vi "Compare Two Paths - Path2 Array.vi"(4 "path2":path[](array[path]), 5 "path1":path) -> (0 "any different types?":bool, 1 "relative path from 1 to 2":path[](array[path]), 2 "common path":path[](array[path]))   [LabVIEW 2020, in "openg_file.lvlib"]
doc: "Compare Two Paths.vi - Compares two paths and if the paths are the same type (both absolute or both relative), the relative path between them is returned."
uses:
  openg_file.lvlib
panel:
  # "Compare Two Paths - Path2 Array.vi\n\nCompares two paths and if the paths are the same type (both absolute or both relative), the relative path between them is returned.\n\nPlease visit http://www.OpenG.org to learn about the\nOpen Source LabVIEW software movement.\n\nNOTICE -- YOU MUST LEAVE THIS NOTICE IN PLACE.  PER THE TERMS OF THE LICENSE BELOW, YOU MAY SUBLICENSE THIS SOFTWARE \nIN ANY WAY THAT DOES NOT CONFLICT WITH THIS LICENSE.\n\n### BSD License (http://www.opensource.org/licenses/bsd-license.php) Begin ###\n\nCopyright (c) 2002, Rolf Kalbermatter <rolf.kalbermatter@citeng.com> \nCopyright (c) 2002-2006, Jim Kring <jim@jimkring.com>\nCopyright (c) 2010, Jonathon Green <jg@jgcode.net>\n\nAll rights reserved.\n\nRedistribution and use in source and binary forms, with or without modification, are permitted provided that the following conditions are met:\n\n    * Redistributions of source code must retain the above copyright notice, this list of conditions and the following disclaimer.\n    * Redistributions in binary form must reproduce the above copyright notice, this list of conditions and the following disclaimer in the \n       documentation and/or other materials provided with the distribution.\n    * Neither the name of SciWare, James Kring, Inc., nor the names of its contributors may be used to endorse or promote products derived \n       from this software without specific prior written permission.\n\nTHIS SOFTWARE IS PROVIDED BY THE COPYRIGHT HOLDERS AND CONTRIBUTORS \"AS IS\" AND ANY EXPRESS OR IMPLIED WARRANTIES, \nINCLUDING, BUT NOT LIMITED TO, THE IMPLIED WARRANTIES OF MERCHANTABILITY AND FITNESS FOR A PARTICULAR PURPOSE ARE \nDISCLAIMED. IN NO EVENT SHALL THE COPYRIGHT OWNER OR CONTRIBUTORS BE LIABLE FOR ANY DIRECT, INDIRECT, INCIDENTAL,\n SPECIAL, EXEMPLARY, OR CONSEQUENTIAL DAMAGES (INCLUDING, BUT NOT LIMITED TO, PROCUREMENT OF SUBSTITUTE GOODS OR \nSERVICES; LOSS OF USE, DATA, OR PROFITS; OR BUSINESS INTERRUPTION) HOWEVER CAUSED AND ON ANY THEORY OF LIABILITY, \nWHETHER IN CONTRACT, STRICT LIABILITY, OR TORT (INCLUDING NEGLIGENCE OR OTHERWISE) ARISING IN ANY WAY OUT OF THE USE \nOF THIS SOFTWARE, EVEN IF ADVISED OF THE POSSIBILITY OF SUCH DAMAGE.\n\n### BSD License End ###"
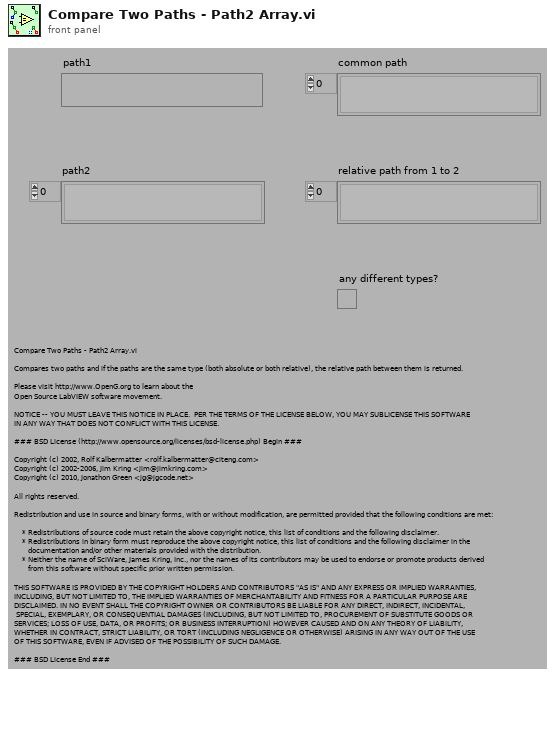
[diagram p1: front panel]
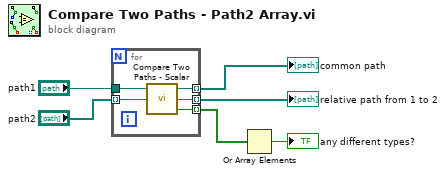
[diagram p0: block diagram]
diagram:
  n1 = for {
    tunnel: [w11] -> w6 mode=indexing
    tunnel: [w10] -> w5 mode=indexing
    tunnel: [w9] -> w4 mode=indexing
    tunnel: "path1" -> [w8]
    tunnel: "path2" -> [w7] mode=indexing
    n2 = call "Compare Two Paths - Scalar.vi"("path2"=w7, "path1"=w8) -> ("different types?"=w11:bool, "relative path from 1 to 2"=w10:path, "common path"=w9:path)  [unwired: 1 in]
  }
  "relative path from 1 to 2" <- w5
  "common path" <- w4
  n3 = Or Array Elements(Boolean array=w6) -> (logical OR=→"any different types?":bool)
